vi "FPGA Run.vi"(6 "stats":i32[](array[numeric]), 7 "runs":i32, 8 "error in (no error)":errorcluster, 9 "fileName":string, 10 "fpgaCommand":u8, 11 "saveClicks":bool) -> (0 "error out":errorcluster, 3 "function return":i32, 4 "stats out":i32[](array[numeric]))   [LabVIEW 2013, in "TimeTagLV.lvlib"]
doc: "LIBRARY_API int FPGA_Run(bool saveClicks, unsigned char fpgaCommand,char* fileName, int* stats, int runs);"
uses:
  TimeTagLV.lvlib
  TimeTag.dll
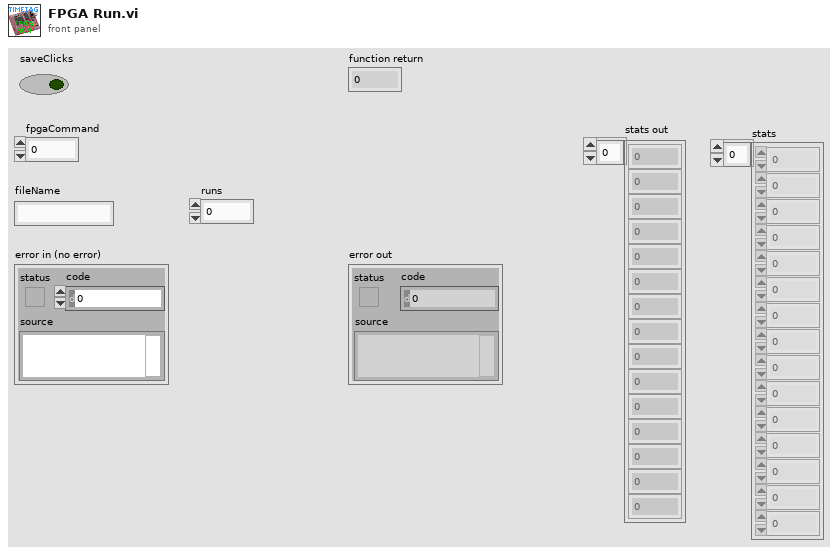
[diagram p1: front panel]
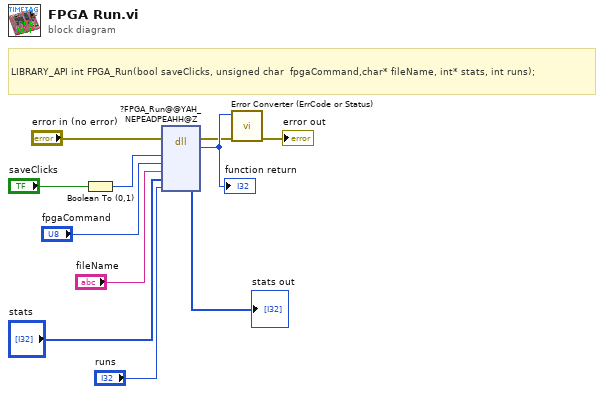
[diagram p0: block diagram]
diagram:
  # "LIBRARY_API int FPGA_Run(bool saveClicks, unsigned char  fpgaCommand,char* fileName, int* stats, int runs);"
  n1 = Boolean To (0,1)(Boolean="saveClicks") -> (0, 1=w9:i16)
  n2 = dll-call lib="C:/FPGA_XyloEM/TimeTagDLL/TimeTagLV/TimeTag.*" fn="?FPGA_Run@@YAH_NEPEADPEAHH@Z"(error in="error in (no error)", "saveClicks"=w9, "fpgaCommand"="fpgaCommand", "fileName"="fileName", "stats"="stats", "runs"="runs") -> (error out=w4:errorcluster, "return type"=w11:i32, "stats"=→"stats out":i32[])  [unwired: 6 in, 1 out]
  "function return" <- w11
  n3 = call "Error Converter (ErrCode or Status).vi"("error in (no error)"=w4, "error code"=w11) -> ("error out"=→"error out":errorcluster)  [unwired: 9 in]
